vi "Get as Boolean.vi"(8 "error in (no error)":errorcluster, 10 "Name Array":string[](array[string]), 11 "JSON Value in":refnum<class "JSON Value.lvclass">) -> (0 "error out":errorcluster, 2 "Boolean":bool, 3 "JSON Value out":refnum<class "JSON Value.lvclass">)   [LabVIEW 2011, in "JSON Scalar.lvclass"]
doc: "Converts a <b>JSON Value</b> into a <b>Boolean</b>.\n't' and 'true' (case insensitive) are converted to a 'TRUE' value.\n\nCopyright 2012 James David Powell, Shaun Rumbell and Ton Plomp\nMore information on http://lavag.org/topic/16217-cr-json-labview"
uses:
  JSON Scalar.lvclass
  JSON Value/JSON Value.lvclass
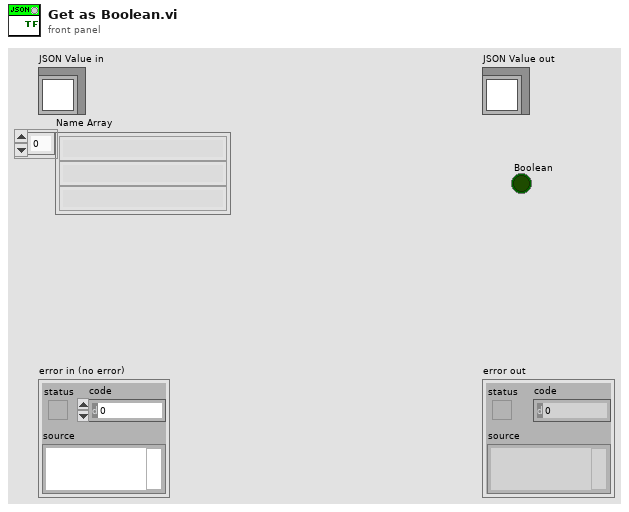
[diagram p1: front panel]
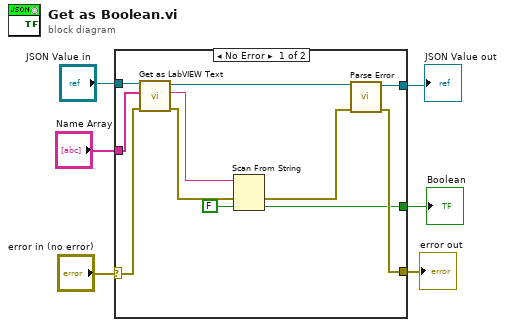
[diagram p0: block diagram]
diagram:
  n1 = case shown="No Error" "error in (no error)" {
    selector: "error in (no error)" -> [w13 w19]
    tunnel: "JSON Value in" -> [w17 w18]
    tunnel: [w15 w18] -> w5
    tunnel: [w14 w19] -> w4
    tunnel: [w9 _] -> w2
    tunnel: "Name Array" -> [w7 _]
    frame No Error {
      n2 = call-dynamic "Get as LabVIEW Text.vi"("error in (no error)"=w13, "Name Array"=w7, "JSON Value In"=w17) -> ("error out"=w11:errorcluster, "LabVIEW Text"=w12:string, "JSON Value Out"=w16:refnum<class "JSON Value.lvclass">)  [unwired: 6 in]
      n3 = Scan From String(input string=w12, error in=w11, default 1=FALSE) -> (error out=w10:errorcluster, output 1=w9:bool)  [unwired: 2 in, 2 out]
      n4 = call-dynamic "Parse Error.vi"("error in (no error)"=w10, "JSON Value in"=w16) -> ("error out"=w14:errorcluster, "JSON Value out"=w15:refnum<class "JSON Value.lvclass">)  [unwired: 8 in]
    }
    frame Error {
    }
  }
  "error out" <- w4
  "JSON Value out" <- w5
  "Boolean" <- w2
